vi "basic-iti.vi"(4 "Cluster":T1, 5 "relative seconds":dbl, 6 "Numeric":dbl, 7 "reference":refnum<vi>, 9 "Period":i64, 10 "reference 2":refnum<vi>, 11 "Cluster in":refnum<vi>) -> (3 "Cluster 2":T1)   [LabVIEW 2015]
uses:
  <vilib>/Platform/TimedLoop/XDataNode/wakeup.ctl
  <vilib>/Platform/TimedLoop/XDataNode/XDNodeRunTimeDep.lvlib
  <vilib>/Platform/TimedLoop/XDataNode/nitl_modes.ctl
  <vilib>/Platform/TimedLoop/XDataNode/timing_clust.ctl
  <vilib>/platform/TimedLoop/XDataNode/XDataNode.xnode
  Device/Methods/Lickometer-Read.vi
  Rack/Methods/Rack-Refresh.vi
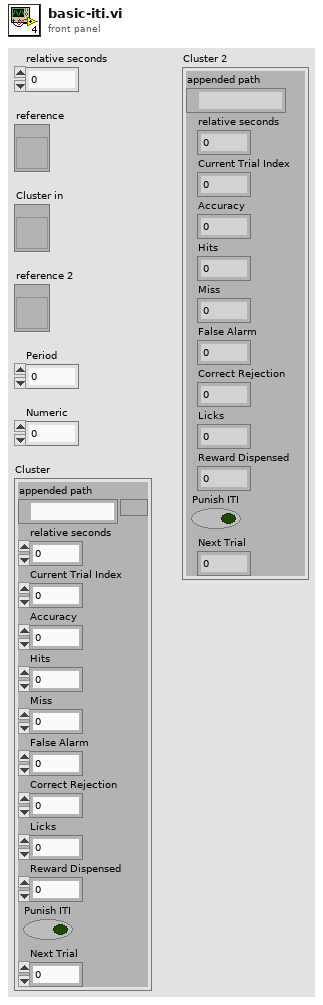
[diagram p1: front panel]
types:
  T1 = cluster{"appended path":path, "relative seconds":dbl, "Current Trial Index":i32, "Accuracy":dbl, "Hits":i32, "Miss":i32, "False Alarm":i32, "Correct Rejection":i32, "Licks":i32, "Reward Dispensed":dbl, "Punish ITI":bool, "Next Trial":i32}
  T2 = typedef "XDNodeRunTimeDep.lvlib/timing_clust.ctl" = cluster{"Expected End [f-1]":u64, "Actual End [f-1]":u64, "Finished Late? [f-1]":bool, "Expected End [i-1]":u64, "Actual End [i-1]":u64, "Finished Late? [i-1]":bool, "Expected Start [i]":u64, "Actual Start [i]":u64, "Expected Start [f]":u64, "Actual Start [f]":u64, "Source Name":string, "Structure Name":string, "Period":i64, "Deadline":i64, "Offset":i64, "Start":i64, "Priority":i32, "Timeout":i32, "Mode":T3, "Wakeup Reason":T4, "Error":errorcluster, "Source Type":string, "Secondary Source Type":string, "Global End Time":u64, "Global Start Time":u64, "Frame Duration":u64, "Iteration Duration":u64, "Assigned CPU":i32, "I/O Scan Engine Mode":u32}
  T3 = typedef "XDNodeRunTimeDep.lvlib/nitl_modes.ctl" = enum32{"No Change", "Process missed periods, maintain original phase", "Discard missed periods, maintain original phase", "Process missed periods, ignore original phase", "Discard missed periods, ignore original phase"}
  T4 = typedef "XDNodeRunTimeDep.lvlib/wakeup.ctl" = enum32{"Normal", "Aborted", "Asynchronous wakeup", "Timing source error", "Timed loop error", "Timeout"}
  T5 = typedef "InputData cluster.ctl" = cluster{"DigitalInput":T6}
  T6 = typedef "DigitalInput-DataCluster.ctl" = cluster{"Falling":bool[], "Rising":bool[], "State":bool[]}
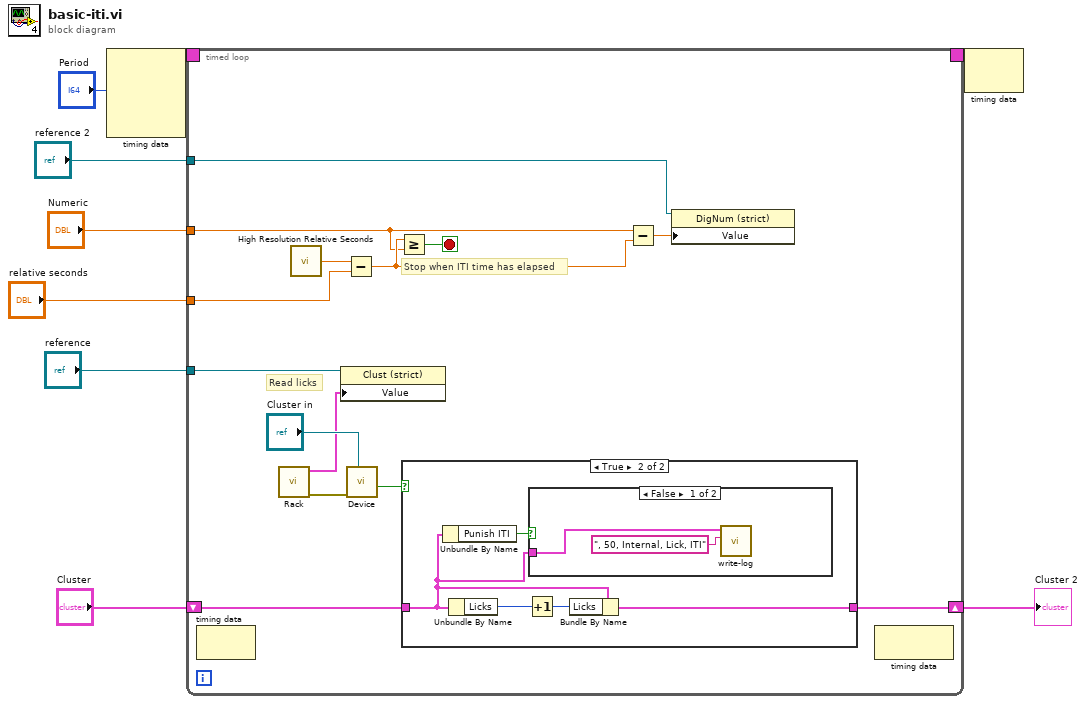
[diagram p0: block diagram]
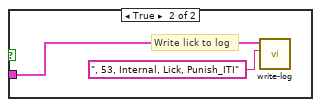
[diagram p3: hidden frame]
diagram:
  n1 = node-c288("Period") -> (w9:T2)  [unwired: 3 in]
  n2 = timed-loop {
    tunnel: "Numeric" -> [w17]
    tunnel: "relative seconds" -> [w18]
    shift-right: [w20] -> w3
    shift-left: "Cluster" -> [w21]
    timing: w9 -> [_]
    timing-out: [_] -> w8
    tunnel: "reference" -> [w11]
    tunnel: "reference 2" -> [w10]
    stop <- w22 stop-if-true
    # "Read licks"
    # "Stop when ITI time has elapsed"
    n3 = node-c288() -> ()  [unwired: 1 in, 1 out]
    n4 = call-poly "Rack.vi"() -> ("error out"=w15:errorcluster, "Data Cluster"=w13:T5)  [unwired: 10 in]
    n5 = call <vilib>:"High Resolution Relative Seconds.vi"() -> ("relative seconds"=w23:dbl)
    n6 = property class="Clust (strict)"(reference=w11, "Value"=w13) -> ()  [unwired: 1 in, 2 out]
    n7 = Subtract(x=w23, y=w18) -> (x-y=w19:dbl)
    n8 = call-poly "Device.vi"("Device reference"="Cluster in", "error in (no error)"=w15) -> ("Lick start?"=w14:bool)  [unwired: 7 in, 2 out]
    n9 = Greater Or Equal?(x=w19, y=w17) -> (x >= y?=w22:bool)
    n10 = case shown="True" w14 {
      tunnel: w21 -> [w26 w27]
      tunnel: [w26 w29] -> w20
      frame False {
      }
      frame True {
        n11 = Unbundle By Name(w27) -> ("Punish ITI"=w28:bool)
        n12 = Unbundle By Name(w27) -> ("Licks"=w31:i32)
        n13 = Increment(x=w31) -> (x+1=w30:i32)
        n14 = case shown="False" w28 {
          tunnel: w27 -> [w33 w34]
          frame False {
            n15 = call "write-log.vi"("Write Text"=", 50, Internal, Lick, ITI" ("text"), "Internal Cluster"=w33) -> ()  [unwired: 10 in]
          }
          frame True {
            # "Write lick to log"
            n16 = call "write-log.vi"("Write Text"=", 53, Internal, Lick, Punish_ITI" ("text"), "Internal Cluster"=w34) -> ()  [unwired: 10 in]
          }
        }
        n17 = Bundle By Name(cluster=w27, "Licks"=w30) -> (w29:T1)
      }
    }
    n18 = Subtract(x=w17, y=w19) -> (x-y=w12:dbl)
    n19 = property class="DigNum (strict)"(reference=w10, "Value"=w12) -> ()  [unwired: 1 in, 2 out]
    n20 = node-c288() -> ()  [unwired: 1 in, 1 out]
  }
  "Cluster 2" <- w3
  n21 = node-c288(w8) -> ()  [unwired: 1 out]
